vi "Open Limit Switch.vi"(2 "DIO Channel":T1, 3 "refnum name":string="My Switch RefNum") -> ()   [LabVIEW 2015]
uses:
  <vilib>/Rock Robotics/SystemInterfaces/DIO/FPGA_DIOChannel.ctl
  <vilib>/Rock Robotics/WPI/Switch/WPI_SwitchOpenLimit.vi
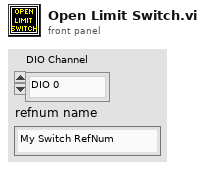
[diagram p1: front panel]
types:
  T1 = typedef "FPGA_DIOChannel.ctl" = enum8{"DIO 0", "DIO 1", "DIO 2", "DIO 3", "DIO 4", "DIO 5", "DIO 6", "DIO 7", "DIO 8", "DIO 9", "DIO MXP 0", "DIO MXP 1", "DIO MXP 2", "DIO MXP 3", "DIO MXP 4", "DIO MXP 5", "DIO MXP 6", "DIO MXP 7", "DIO MXP 8", "DIO MXP 9", "DIO MXP 10", "DIO MXP 11", "DIO MXP 12", "DIO MXP 13", "DIO MXP 14", "DIO MXP 15", "Invalid"}
  T2 = typedef "WPI_SwitchDevRef.ctl" = cluster{"DevStatus":errorcluster, "DIO Channel":T1, "CntIndex":T3, "Normally Closed":bool}
  T3 = typedef "FPGA_CounterCtrSystemIndex.ctl" = enum8{"Ctr 0", "Ctr 1", "Ctr 2", "Ctr 3", "Ctr 4", "Ctr 5", "Ctr 6", "Ctr 7", "Invalid"}
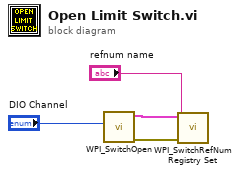
[diagram p0: block diagram]
diagram:
  n1 = call-poly <vilib>:"WPI_SwitchOpen.vi"("DIO Channel"="DIO Channel") -> ("error out"=w2:errorcluster, "SwitchDevRef"=w3:T2)  [unwired: 9 in]
  n2 = call <vilib>:"WPI_SwitchRefNum Registry Set.vi"("error in (no error)"=w2, "refnum name"="refnum name", "SwitchDevRef"=w3) -> ()  [unwired: 7 in, 2 out]
